vi "SDG60ConfSTDWFM.vi"(0 "VISA resource name":refnum<visa-resource-name>="USB0::0xF4EC::0x1101::SDG6XEBC5R0119::INSTR", 1 "Frequency/Period (1 Hz/s)":dbl=2.0 format="%#.16g", 2 "DC Offset (0.00 V)":dbl format="%#_15g", 5 "Channel (1:Channel 1)":i32(ring)=1 items=["Channel 1"=1, "Channel 2"=2], 7 "Waveform Function (0: Sine)":u16(ring) items=["Sine", "Square", "Ramp", "DC", "Pulse", "Arb"], 9 "Amplitude (1.0 Vpp)":dbl=0.1 format="%#.6f", 11 "Phase (0.0 degrees)":dbl min=-360.0 max=360.0 format="%#.15g", 12 "Symmetry/Duty (50.0 %)":dbl=50.0 format="%#.6f", 13 "Freq/Period (T:Freq)":bool=TRUE) -> (4 "VISA resource name out":refnum<visa-resource-name>, 15 "error out":errorcluster)   [LabVIEW 2018]
doc: "Selects the waveform shape, frequency, amplitude, offset, and phase for standard waveforms (including Sine, Square, Ramp, Pulse, DC and Arb).\n\nNotes: \nTo configure other parameters for pulse waveforms please run the Configure Pulse VI. \nTo configure noise waveform please run the Configure Noise VI.\nTo configure other parameters for arbitrary waveforms please run the Create Arbitrary Waveform. \nTo configure PRBS waveform please run the Configure PRBS Waveform VI."
panel:
  in  "error in (no error)":errorcluster
  # "For Noise use seperate vi\nFor ARB, must follow up with SDG60ConfArbWaveform.\nIf using user ARB, precede with SDG60CreateArbWaveform.\nFor pulse must follow up with seperate vi to change parameters (in fact don't need this vi to set pulses at all)"
  # "0.1mV resolution"
  # "Range: 1 uHz-200 MHz  (Sine)\nRange: 20 ns-1 Ms\nInternal setting max res 10 digits for freq, 6 digits for period"
  # "Ignored for all but Ramp and Square\nSymmetry range :0%-100%\nDuty range: 0.001%-Max depends on freq\n6 digit precision (~73..99%)"
  # "0.1mV resolution"
  # "Res: 0.001 degree. Range +/-279 deg"
  # "Operating sequence in case output is already on:\nWhen run, will turn off output for ~150ms\nthen turn use set waveform\nthen freq change\nthen amp change\nthen use DC offset\nthen use phase offset (discontiouse)"
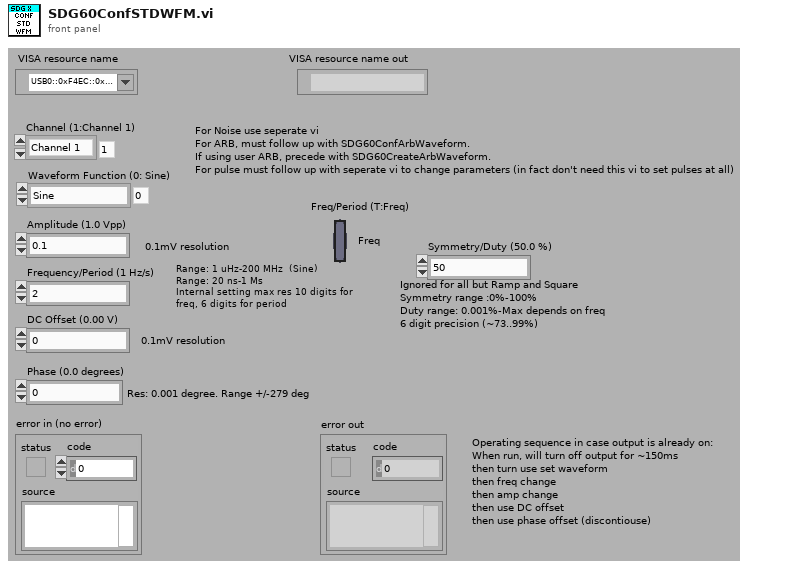
[diagram p1: front panel]
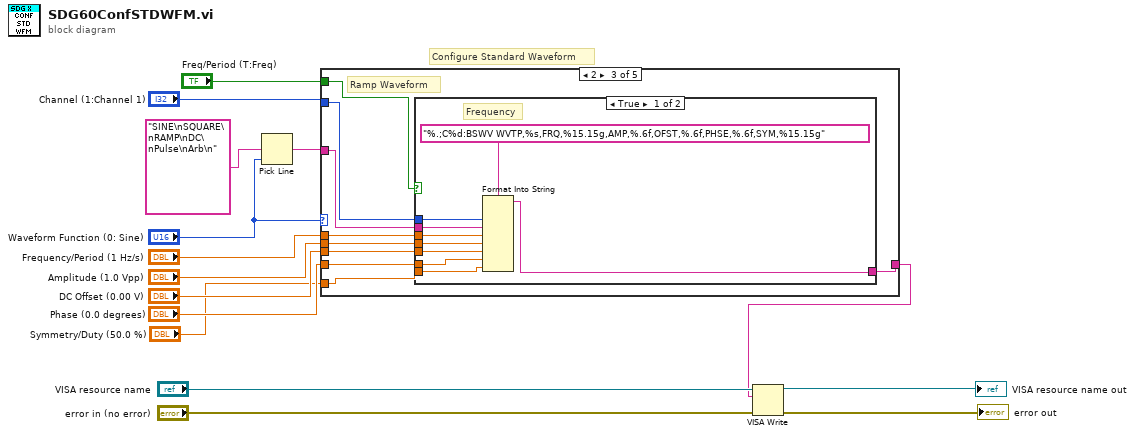
[diagram p0: block diagram]
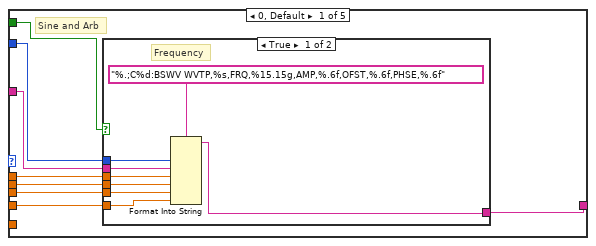
[diagram p2: hidden frame]
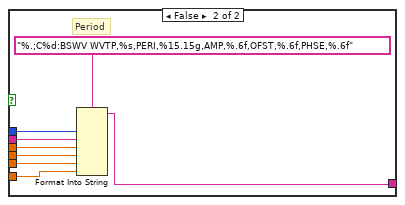
[diagram p3: hidden frame]
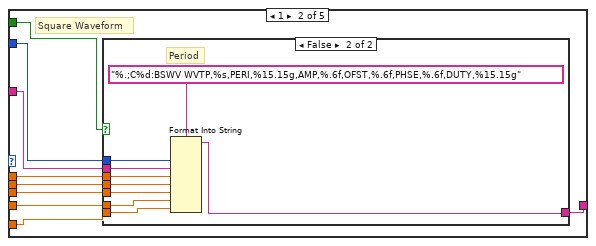
[diagram p4: hidden frame]
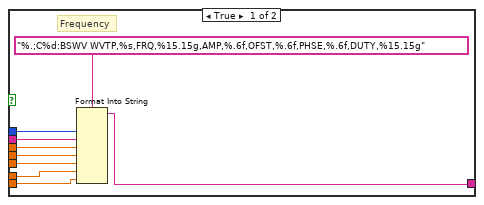
[diagram p5: hidden frame]
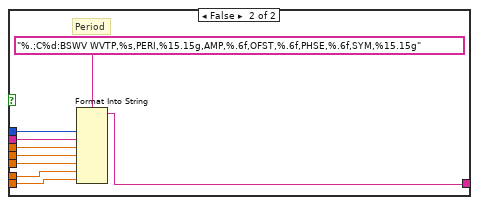
[diagram p6: hidden frame]
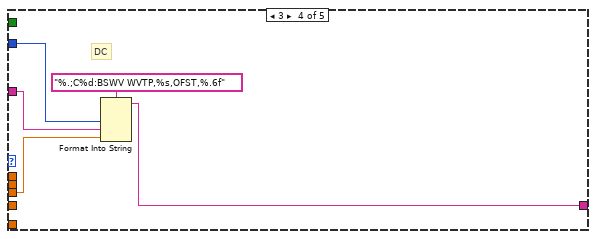
[diagram p7: hidden frame]
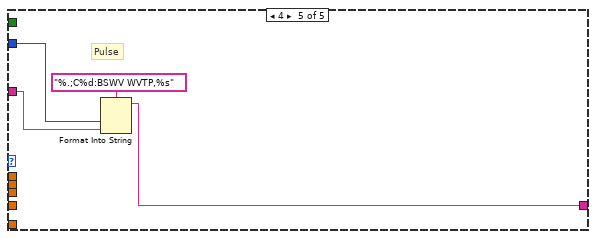
[diagram p8: hidden frame]
diagram:
  # "Configure Standard Waveform"
  n1 = Pick Line(multi-line string="SINE\nSQUARE\nRAMP\nDC\nPulse\nArb\n", line index="Waveform Function (0: Sine)") -> (output string=w14:string)  [unwired: 1 in]
  n2 = case shown="2" "Waveform Function (0: Sine)" {
    tunnel: w14 -> [w23 w48 w75 w96 w100]
    tunnel: [w22 w47 w74 w94 w99] -> w11
    tunnel: "Phase (0.0 degrees)" -> [w21 w46 w73 _ _]
    tunnel: "DC Offset (0.00 V)" -> [w20 w45 w72 w95 _]
    tunnel: "Amplitude (1.0 Vpp)" -> [w19 w44 w71 _ _]
    tunnel: "Frequency/Period (1 Hz/s)" -> [w18 w43 w70 _ _]
    tunnel: "Channel (1:Channel 1)" -> [w17 w42 w69 w97 w101]
    tunnel: "Freq/Period (T:Freq)" -> [w16 w41 w68 _ _]
    tunnel: "Symmetry/Duty (50.0 %)" -> [_ w40 w67 _ _]
    frame 0, Default {
      # "Sine and Arb"
      n3 = case shown="True" w16 {
        tunnel: w23 -> [w31 w39]
        tunnel: [w29 w37] -> w22
        tunnel: w21 -> [w28 w36]
        tunnel: w20 -> [w27 w35]
        tunnel: w19 -> [w26 w34]
        tunnel: w18 -> [w25 w33]
        tunnel: w17 -> [w24 w32]
        frame True {
          # "Frequency"
          n4 = Format Into String(format string="%.;C%d:BSWV WVTP,%s,FRQ,%15.15g,AMP,%.6f,OFST,%.6f,PHSE,%.6f", w24, w31, w25, w26, w27, w28) -> (resulting string=w29:string)  [unwired: 2 in, 1 out]
        }
        frame False {
          # "Period"
          n5 = Format Into String(format string="%.;C%d:BSWV WVTP,%s,PERI,%15.15g,AMP,%.6f,OFST,%.6f,PHSE,%.6f", w32, w39, w33, w34, w35, w36) -> (resulting string=w37:string)  [unwired: 2 in, 1 out]
        }
      }
    }
    frame 1 {
      # "Square Waveform"
      n6 = case shown="False" w41 {
        tunnel: w48 -> [w57 w66]
        tunnel: [w55 w64] -> w47
        tunnel: w46 -> [w54 w63]
        tunnel: w45 -> [w53 w62]
        tunnel: w44 -> [w52 w61]
        tunnel: w43 -> [w51 w60]
        tunnel: w42 -> [w50 w59]
        tunnel: w40 -> [w49 w58]
        frame True {
          # "Frequency"
          n7 = Format Into String(format string="%.;C%d:BSWV WVTP,%s,FRQ,%15.15g,AMP,%.6f,OFST,%.6f,PHSE,%.6f,DUTY,%15.15g", w50, w57, w51, w52, w53, w54, w49) -> (resulting string=w55:string)  [unwired: 2 in, 1 out]
        }
        frame False {
          # "Period"
          n8 = Format Into String(format string="%.;C%d:BSWV WVTP,%s,PERI,%15.15g,AMP,%.6f,OFST,%.6f,PHSE,%.6f,DUTY,%15.15g", w59, w66, w60, w61, w62, w63, w58) -> (resulting string=w64:string)  [unwired: 2 in, 1 out]
        }
      }
    }
    frame 2 {
      # "Ramp Waveform"
      n9 = case shown="True" w68 {
        tunnel: w75 -> [w84 w93]
        tunnel: [w82 w91] -> w74
        tunnel: w73 -> [w81 w90]
        tunnel: w72 -> [w80 w89]
        tunnel: w71 -> [w79 w88]
        tunnel: w70 -> [w78 w87]
        tunnel: w69 -> [w77 w86]
        tunnel: w67 -> [w76 w85]
        frame True {
          # "Frequency"
          n10 = Format Into String(format string="%.;C%d:BSWV WVTP,%s,FRQ,%15.15g,AMP,%.6f,OFST,%.6f,PHSE,%.6f,SYM,%15.15g", w77, w84, w78, w79, w80, w81, w76) -> (resulting string=w82:string)  [unwired: 2 in, 1 out]
        }
        frame False {
          # "Period"
          n11 = Format Into String(format string="%.;C%d:BSWV WVTP,%s,PERI,%15.15g,AMP,%.6f,OFST,%.6f,PHSE,%.6f,SYM,%15.15g", w86, w93, w87, w88, w89, w90, w85) -> (resulting string=w91:string)  [unwired: 2 in, 1 out]
        }
      }
    }
    frame 3 {
      # "DC"
      n12 = Format Into String(format string="%.;C%d:BSWV WVTP,%s,OFST,%.6f", w97, w96, w95) -> (resulting string=w94:string)  [unwired: 2 in, 1 out]
    }
    frame 4 {
      # "Pulse"
      n13 = Format Into String(format string="%.;C%d:BSWV WVTP,%s", w101, w100) -> (resulting string=w99:string)  [unwired: 2 in, 1 out]
    }
  }
  n14 = VISA Write(VISA resource name="VISA resource name", write buffer=w11, error in (no error)="error in (no error)") -> (VISA resource name out=→"VISA resource name out":refnum<visa-resource-name>, error out=→"error out":errorcluster)  [unwired: 1 out]
